vi "change alias and editor properties.vi"(8 "error in":errorcluster, 10 "default node":refnum<class "NISE_CEF_serializable node.lvclass">, 11 "PL_System Configuration in":refnum<class "NISE_CEF_serializable configuration.lvclass">) -> (0 "error out":errorcluster, 3 "PL_System Configuration out":refnum<class "NISE_CEF_serializable configuration.lvclass">)   [LabVIEW 2013]
uses:
  <vilib>/NI/Configuration Framework/serializable configuration/NISE_CEF_serializable configuration.lvclass
  <vilib>/NI/Configuration Framework/serializable node/NISE_CEF_serializable node.lvclass
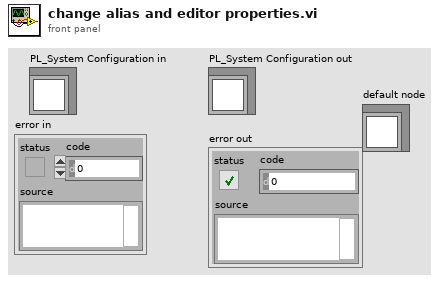
[diagram p1: front panel]
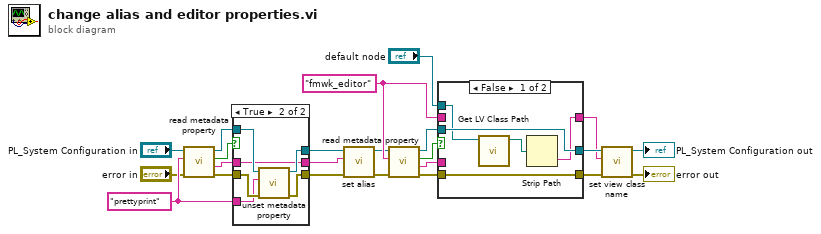
[diagram p0: block diagram]
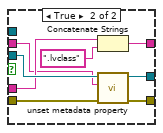
[diagram p2: hidden frame]
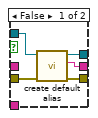
[diagram p3: hidden frame]
diagram:
  w22 = "prettyprint" ("key")
  w21 = "fmwk_editor" ("key")
  n1 = call <vilib>:"read metadata property.vi"("error in"="error in", "key"=w22, "configuration in"="PL_System Configuration in") -> ("error out"=w13:errorcluster, "value"=w23:string, "found"=w17:bool, "configuration out"=w12:refnum<class "NISE_CEF_serializable configuration.lvclass">)  [unwired: 5 in]
  n2 = case shown="True" w17 {
    tunnel: w12 -> [w28 w34]
    tunnel: w13 -> [w27 w33]
    tunnel: [w26 w30] -> w8
    tunnel: [w25 w31] -> w14
    tunnel: w22 -> [_ w32]
    tunnel: w23 -> [_ w29]
    tunnel: [w24 w29] -> w6
    frame False {
      n3 = call-dynamic "create default alias.vi"("error in"=w27, "configuration in"=w28) -> ("error out"=w25:errorcluster, "default alias"=w24:string, "configuration out"=w26:refnum<class "NISE_CEF_serializable configuration.lvclass">)  [unwired: 7 in]
    }
    frame True {
      n4 = call <vilib>:"unset metadata property.vi"("error in"=w33, "key"=w32, "configuration in"=w34) -> ("error out"=w31:errorcluster, "configuration out"=w30:refnum<class "NISE_CEF_serializable configuration.lvclass">)  [unwired: 7 in]
    }
  }
  n5 = call <vilib>:"set alias.vi"("error in"=w14, "alias"=w6, "configuration in"=w8) -> ("error out"=w9:errorcluster, "configuration out"=w7:refnum<class "NISE_CEF_serializable configuration.lvclass">)  [unwired: 7 in]
  n6 = call <vilib>:"read metadata property.vi"("error in"=w9, "key"=w21, "configuration in"=w7) -> ("error out"=w16:errorcluster, "value"=w20:string, "found"=w19:bool, "configuration out"=w15:refnum<class "NISE_CEF_serializable configuration.lvclass">)  [unwired: 5 in]
  n7 = case shown="False" w19 {
    tunnel: w15 -> [w39 w47]
    tunnel: w16 -> [w38 w46]
    tunnel: [w38 w42] -> w18
    tunnel: [w39 w41] -> w4
    tunnel: w20 -> [_ w45]
    tunnel: w21 -> [_ w43]
    tunnel: [w35 w40] -> w2
    tunnel: "default node" -> [w37 _]
    frame False {
      n8 = call <vilib>:"Get LV Class Path.vi"("object"=w37) -> ("class path"=w36:path)  [unwired: 9 in, 1 out]
      n9 = Strip Path(path=w36) -> (name=w35:string)  [unwired: 1 out]
    }
    frame True {
      n10 = Concatenate Strings(w45, ".lvclass" ("string")) -> (w40:string)
      n11 = call <vilib>:"unset metadata property.vi"("error in"=w46, "key"=w43, "configuration in"=w47) -> ("error out"=w42:errorcluster, "configuration out"=w41:refnum<class "NISE_CEF_serializable configuration.lvclass">)  [unwired: 7 in]
    }
  }
  n12 = call <vilib>:"set view class name.vi"("error in"=w18, "view class"=w2, "configuration in"=w4) -> ("error out"=→"error out":errorcluster, "configuration out"=→"PL_System Configuration out":refnum<class "NISE_CEF_serializable configuration.lvclass">)  [unwired: 7 in]
